vi "Initialize UI.vi"(0 "Room Service Manager UI in":refnum<class "Room Service Manager UI.lvclass">, 11 "error in (no error)":errorcluster) -> (4 "Room Service Manager UI out":refnum<class "Room Service Manager UI.lvclass">, 15 "error out":errorcluster)   [LabVIEW 2023, in "Room Service Manager UI.lvlib" / "Room Service Manager UI.lvclass"]
uses:
  Room Service Manager UI.lvclass
  Room Service Manager UI.lvclass/Room Service Manager UI.ctl
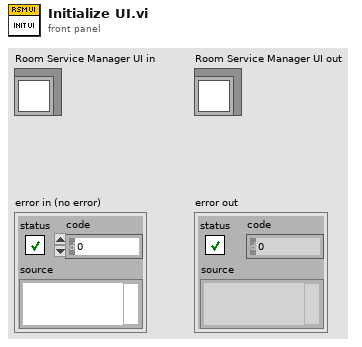
[diagram p1: front panel]
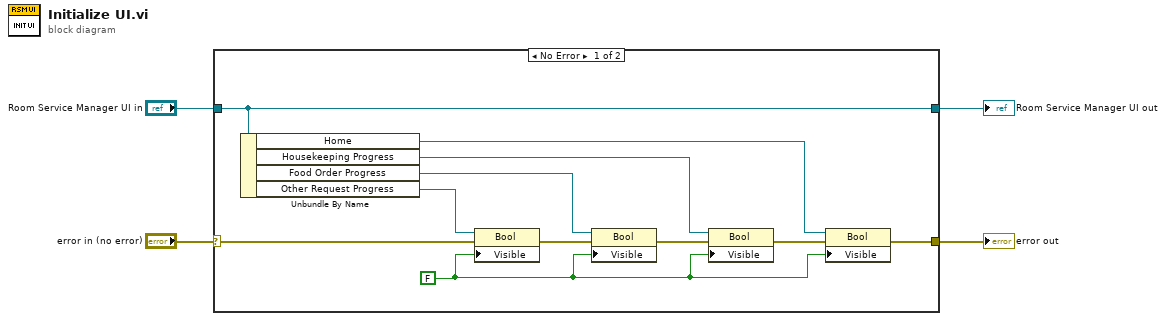
[diagram p0: block diagram]
diagram:
  n1 = case shown="No Error" "error in (no error)" {
    selector: "error in (no error)" -> [w12 w17]
    tunnel: [w13 w17] -> w3
    tunnel: [w15 w16] -> w1
    tunnel: "Room Service Manager UI in" -> [w15 w16]
    frame No Error {
      w8 = FALSE ("Visible")
      n2 = Unbundle By Name(w15) -> ("Home"=w14:refnum<vi>, "Housekeeping Progress"=w5:refnum<vi>, "Food Order Progress"=w6:refnum<vi>, "Other Request Progress"=w7:refnum<vi>)
      n3 = property class="Bool"(reference=w7, error in=w12, "Visible"=w8) -> (error out=w11:errorcluster)  [unwired: 1 out]
      n4 = property class="Bool"(reference=w6, error in=w11, "Visible"=w8) -> (error out=w10:errorcluster)  [unwired: 1 out]
      n5 = property class="Bool"(reference=w5, error in=w10, "Visible"=w8) -> (error out=w9:errorcluster)  [unwired: 1 out]
      n6 = property class="Bool"(reference=w14, error in=w9, "Visible"=w8) -> (error out=w13:errorcluster)  [unwired: 1 out]
    }
    frame Error {
    }
  }
  "error out" <- w3
  "Room Service Manager UI out" <- w1
